vi "FirmaDAQ.vi"() -> ()   [LabVIEW 2016]
uses:
  <vilib>/Utility/miscctls.llb/LVMouseTypeDef.ctl
  <vilib>/DAQmx/write.llb/DAQmx Write (Analog 2D DBL NChan NSamp).vi
  <vilib>/DAQmx/create/channels.llb/DAQmx Create Channel (AO-Voltage-Basic).vi
  <vilib>/DAQmx/configure/timing.llb/DAQmx Timing (Sample Clock).vi
  <vilib>/DAQmx/miscellaneous.llb/DAQmx Fill In Error Info.vi
panel:
  in  "Stop Button 2":bool
  out "number of samples written per channel":u32
  out "XY Graph":cluster{dbl[], dbl[]}(graph)
  out "2D Picture":picture
  in  "Presentar":bool
  out "Mouse":T1
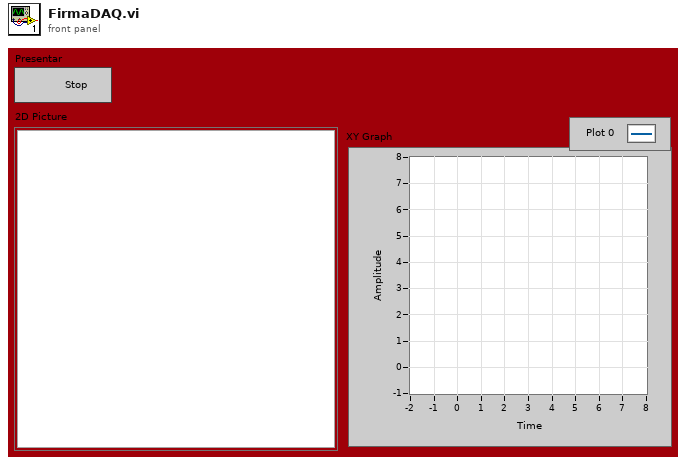
[diagram p1: front panel]
types:
  T1 = typedef "LVMouseTypeDef.ctl" = cluster{"Mouse Position":cluster{"X":i32, "Y":i32}, "Mouse Modifiers":cluster{"Button Down":bool, "Shift Mod":bool, "Menu Mod":bool, "Option Mod":bool}}
  T2 = cluster{"Width":u16, "Style":enum32{"Solid", "Dash", "Dot", "DashDot", "DashDotDot"}}
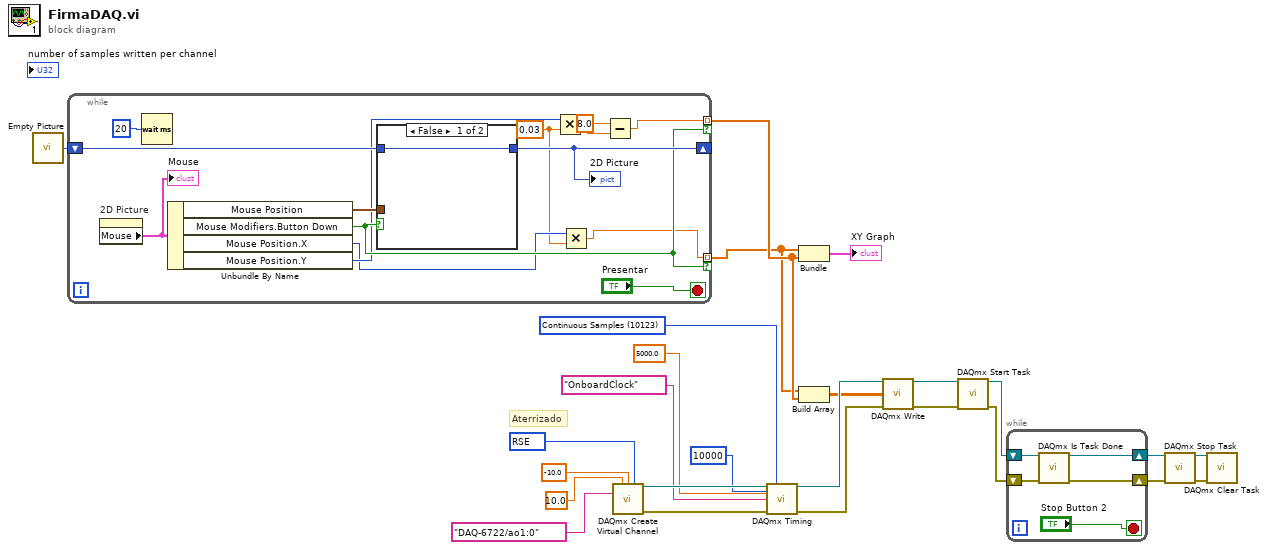
[diagram p0: block diagram]
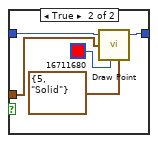
[diagram p2: hidden frame]
diagram:
  w3 = 10123 items=["Finite Samples"=10178, "Continuous Samples"=10123, "Hardware Timed Single Point"=12522] ("sample mode")
  w21 = 10083 items=["Default"=-1, "RSE"=10083, "NRSE"=10078, "Differential"=10106, "Pseudodifferential"=12529] ("input terminal configuration")
  # "Aterrizado"
  n1 = call "Empty Picture"() -> ("empty picture"=w25:picture)
  n2 = while {
    shift-right: [w37] -> _
    shift-left: w25 -> [w36]
    tunnel: [w29] -> w1 mode=indexing if=w33
    tunnel: [w26] -> w2 mode=indexing if=w33
    stop <- "Presentar" stop-if-true
    w30 = 0.03 ("y")
    n3 = property on="2D Picture" class="Pict"() -> ("Mouse"=w35:T1)  [unwired: 2 in, 2 out]
    "Mouse" <- w35
    n4 = Wait (ms)(milliseconds to wait=u32 20) -> ()  [unwired: 1 out]
    n5 = Unbundle By Name(w35) -> ("Mouse Position"=w34:cluster{"X":i32, "Y":i32}, "Mouse Modifiers.Button Down"=w33:bool, "Mouse Position.X"=w31:i32, "Mouse Position.Y"=w32:i32)
    n6 = case shown="False" w33 {
      tunnel: [w40 w43] -> w37
      tunnel: w36 -> [w40 w42]
      tunnel: w34 -> [_ w41]
      frame False {
      }
      frame True {
        n7 = call <vilib>:"Draw Point.vi"("picture"=w42, "point(x,y)"=w41, "color(black)"=u32 16711680, "pen"=T2 {"Width"=5, "Style"=enum."Solid"}) -> ("new picture"=w43:picture)  [unwired: 5 in]
      }
    }
    "2D Picture" <- w37
    n8 = Multiply(x=w32, y=w30) -> (x*y=w27:dbl)
    n9 = Multiply(x=w31, y=w30) -> (x*y=w29:dbl)
    n10 = Subtract(x=8.0, y=w27) -> (x-y=w26:dbl)
  }
  n11 = call-poly <vilib>:"DAQmx Create Virtual Channel.vi"("maximum value"=10.0, "minimum value"=-10.0, "output terminal configuration"=w21, "physical channels"=tag "DAQ-6722/ao1:0") -> ("task out"=w17:refnum<k21>, "error out"=w16:errorcluster)  [unwired: 10 in]
  n12 = call-poly <vilib>:"DAQmx Timing.vi"("task/channels in"=w17, "sample mode"=w3, "samples per channel"=10000, "rate"=5000.0, "source"=tag "OnboardClock", "error in"=w16) -> ("task out"=w12:refnum<k21>, "error out"=w11:errorcluster)  [unwired: 8 in]
  n13 = Bundle(w1, w2) -> (→"XY Graph":cluster{dbl[], dbl[]})  [unwired: 1 in]
  n14 = Build Array(w1, w2) -> (w4:dbl[][])
  n15 = call-poly <vilib>:"DAQmx Write.vi"("task/channels in"=w12, "data"=w4, "error in"=w11) -> ("task out"=w10:refnum<k21>, "error out"=w9:errorcluster)  [unwired: 10 in, 1 out]
  n16 = call <vilib>:"DAQmx Start Task.vi"("task/channels in"=w10, "error in"=w9) -> ("task out"=w8:refnum<k21>, "error out"=w7:errorcluster)  [unwired: 12 in]
  n17 = while {
    shift-right: [w48] -> w6
    shift-left: w8 -> [w50]
    shift-right: [w47] -> w5
    shift-left: w7 -> [w49]
    stop <- "Stop Button 2" stop-if-true
    n18 = call <vilib>:"DAQmx Is Task Done.vi"("task/channels in"=w50, "error in"=w49) -> ("task out"=w48:refnum<k21>, "error out"=w47:errorcluster)  [unwired: 11 in, 1 out]
  }
  n19 = call <vilib>:"DAQmx Stop Task.vi"("task/channels in"=w6, "error in"=w5) -> ("task out"=w20:refnum<k21>, "error out"=w19:errorcluster)  [unwired: 12 in]
  n20 = call <vilib>:"DAQmx Clear Task.vi"("task in"=w20, "error in"=w19) -> ()  [unwired: 13 in, 1 out]
